vi "Data.vi"(7 "LWSR":refnum<class "Web Request.lvclass">) -> ()   [LabVIEW 2015]
uses:
  <vilib>/wsapi/Web Request.lvclass
panel:
  out "resulting string":string
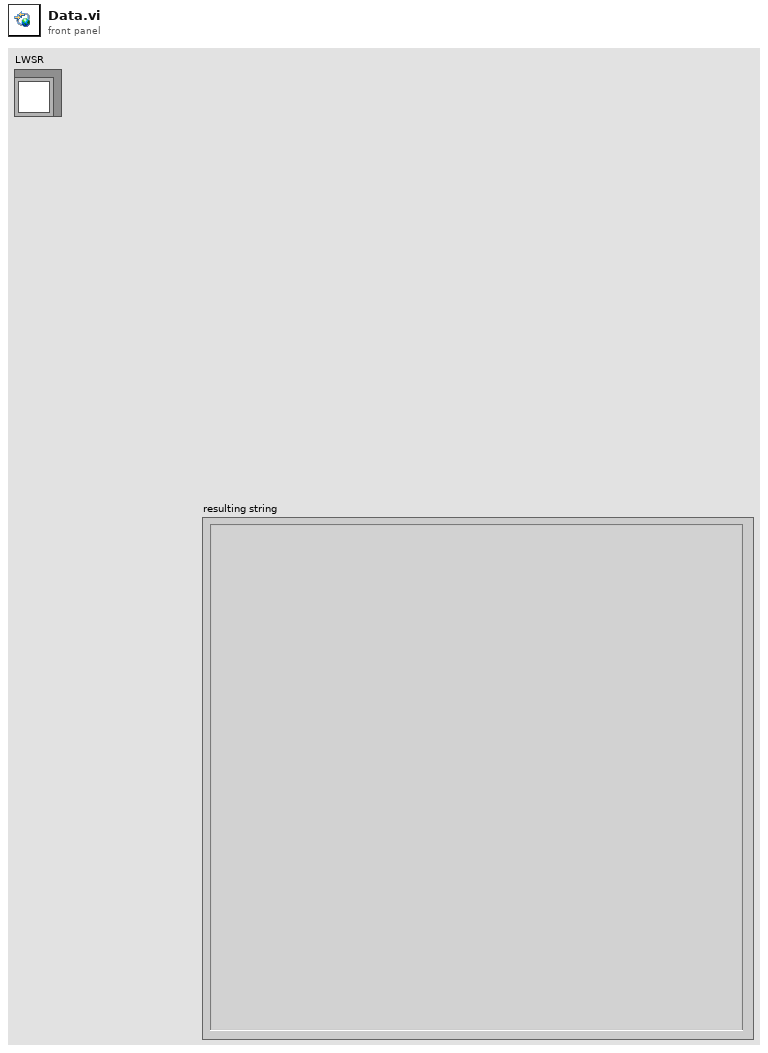
[diagram p1: front panel]
types:
  T1 = typedef "Data.ctl" = cluster{"Voltage":dbl, "Amperage":dbl, "Wattage":dbl, "Power Factor":dbl, "Voltage Distortion":dbl, "Amperage Distortion":dbl}
  T2 = cluster{"Power Data":T1[], "Time":timestamp, "Temperature":dbl}
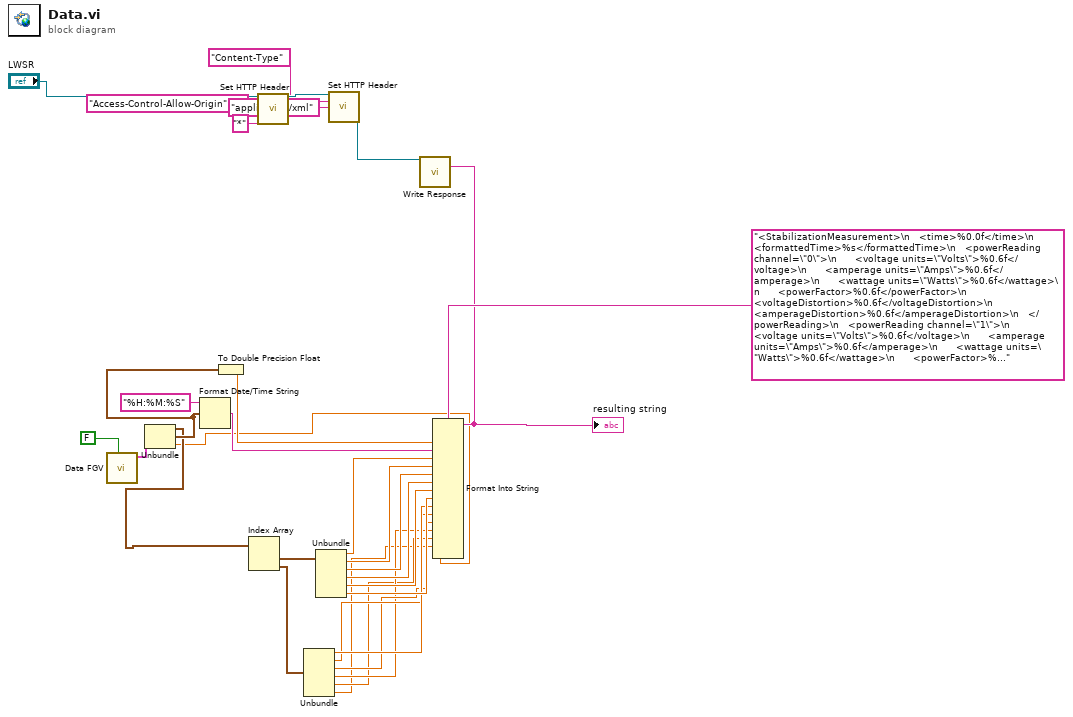
[diagram p0: block diagram]
diagram:
  n1 = call "Data FGV.vi"("Write?"=FALSE) -> ("Data Out"=w27:T2)  [unwired: 10 in]
  n2 = Unbundle(w27) -> ("Power Data"=w16:T1[], "Time"=w18:timestamp, "Temperature"=w1:dbl)
  n3 = Format Date/Time String(time format string (%c)="%H:%M:%S", seconds (now)=w18) -> (date/time string=w29:string)  [unwired: 1 in]
  n4 = To Double Precision Float(number=w18) -> (double precision float=w17:dbl)
  n5 = Index Array(array=w16) -> (element #1=w15:T1, element #2=w8:T1)  [unwired: 2 in]
  n6 = call <vilib>:"Set HTTP Header.vi"("LabVIEW Web Service Request"="LWSR", "header"="Access-Control-Allow-Origin", "header value"="*") -> ("LabVIEW Web Service Request out"=w22:refnum<class "Web Request.lvclass">)  [unwired: 11 in, 1 out]
  n7 = Unbundle(w8) -> ("Voltage"=w7:dbl, "Amperage"=w6:dbl, "Wattage"=w5:dbl, "Power Factor"=w4:dbl, "Voltage Distortion"=w3:dbl, "Amperage Distortion"=w2:dbl)
  n8 = Unbundle(w15) -> ("Voltage"=w14:dbl, "Amperage"=w13:dbl, "Wattage"=w12:dbl, "Power Factor"=w11:dbl, "Voltage Distortion"=w10:dbl, "Amperage Distortion"=w9:dbl)
  n9 = call <vilib>:"Set HTTP Header.vi"("LabVIEW Web Service Request"=w22, "header"="Content-Type", "header value"="application/xml") -> ("LabVIEW Web Service Request out"=w21:refnum<class "Web Request.lvclass">)  [unwired: 11 in, 1 out]
  n10 = Format Into String(format string="<StabilizationMeasurement>\n   <time>%0.0f</time>\n   <formattedTime>%s</formattedTime>\n   <powerReading channel=\"0\">\n      <voltage units=\"Volts\">%0.6f</voltage>\n      <amperage units=\"Amps\">%0.6f</amperage>\n      <wattage units=\"Watts\">%0.6f</wattage>\n      <powerFactor>%0.6f</powerFactor>\n      <voltageDistortion>%0.6f</voltageDistortion>\n      <amperageDistortion>%0.6f</amperageDistortion>\n   </powerReading>\n   <powerReading channel=\"1\">\n      <voltage units=\"Volts\">%0.6f</voltage>\n      <amperage units=\"Amps\">%0.6f</amperage>\n      <wattage units=\"Watts\">%0.6f</wattage>\n      <powerFactor>%0.6f</powerFactor>\n      <voltageDistortion>%0.6f</voltageDistortion>\n      <amperageDistortion>%0.6f</amperageDistortion>\n   </powerReading>\n   <temperatureReading channel=\"0\" units=\"degC\">%0.6f</temperatureReading>\n   <temperatureReading>Thermocouple is disconnected</temperatureReading>\n</StabilizationMeasurement>", w17, w29, w14, w13, w12, w11, w10, w9, w7, w6, w5, w4, w3, w2, w1) -> (resulting string=w25:string)  [unwired: 2 in, 1 out]
  "resulting string" <- w25
  n11 = call <vilib>:"Write Response.vi"("LabVIEW Web Service Request"=w21, "response string"=w25) -> ()  [unwired: 12 in, 2 out]
